vi "Boolean to Disable State.vi"(1 "enable?":bool) -> (0 "disable state":T1(ring))   [LabVIEW 2017]
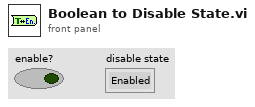
[diagram p1: front panel]
types:
  T1 = enum8{"Enabled", "Disabled", "Disabled and Grayed Out"}
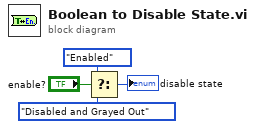
[diagram p0: block diagram]
diagram:
  n1 = Select(t=T1."Enabled" ("Disabled"), s="enable?", f=T1."Disabled and Grayed Out") -> (s? t:f=→"disable state":T1)
